vi "RT Driver VI.vi"(7 "Operation":T1, 11 "Device Reference in":T2 format="%.0x") -> (0 "Error Code":i32)   [LabVIEW 2015, in "J1939 Addon Engine.lvlib"]
uses:
  J1939 Addon Engine.lvlib
  <vilib>/NI Veristand/Custom Device API/Custom Device Item Ref.ctl
  <vilib>/NI Veristand/Custom Device API/Hardware Interface Driver VI Operation.ctl
  <vilib>/NI/NIVS Inline Async API/_VS Inline Async API/VS Inline Async API/VS Inline Async API.lvclass/VS Inline Async API.ctl
  <vilib>/NI/NIVS Inline Async API/_Data Access Engine/Data Access Engine/Data Access Engine.lvclass/Data Access Engine.ctl
  <vilib>/NI/NIVS Inline Async API/_Data Access Engine/Access Type Classes/Write/Write.lvclass/Write.ctl
  <vilib>/NI/NIVS Inline Async API/_Data Access Engine/Access Type Classes/ReadWrite/ReadWrite.lvclass/ReadWrite.ctl
  <vilib>/NI/NIVS Inline Async API/_Data Access Engine/Access Type Classes/Read/Read.lvclass/Read.ctl
  <vilib>/NI/NIVS Inline Async API/_Data Access Engine/Data Access Engine/Methods/Data.Engine.Read Data from HW.vi
  <vilib>/NI/NIVS Inline Async API/_VS Inline Async API/Error Handling Process/SubVIs/Error.GetError.vi
  <vilib>/NI Veristand/Custom Device API/NI VeriStand - Set Channel Values by Block Data Reference.vi
  <vilib>/NI Veristand/Custom Device API/NI VeriStand - Get Channel Values by Block Data Reference.vi
  <vilib>/NI/NIVS Inline Async API/_Data Access Engine/Data Access Engine/Methods/Data.Engine.Write Data to HW.vi
  <vilib>/NI/NIVS Inline Async API/_Data Access Engine/Access Type Classes/ReadWrite/ReadWrite.EngineData.vi
  <vilib>/NI/NIVS Inline Async API/_Data Access Engine/Access Type Classes/Write/Write.EngineData.vi
  <vilib>/NI/NIVS Inline Async API/_Data Access Engine/Access Type Classes/Read/Read.EngineData.vi
  <vilib>/NI Veristand/Custom Device API/NI VeriStand - Get Channel Value by Data Reference.vi
  <vilib>/NI Veristand/Custom Device API/NI VeriStand - Set Channel Value by Data Reference.vi
  SubVIs/Main.Load 986x Bitfile.vi
  SubVIs/Main.InitializeXNET.vi
  <vilib>/NI Veristand/Custom Device API/Global Data Refs.vi
  <vilib>/xnet/xnet.llb/XNET Read.vi
  <vilib>/xnet/xnet.llb/XNET Read (Signal Single-point).vi
  <vilib>/xnet/xnet.llb/XNET Read (Signal XY).vi
  <vilib>/xnet/xnet.llb/XNET Write.vi
  <vilib>/xnet/xnet.llb/XNET Write (Signal Single-point).vi
  <vilib>/xnet/xnet.llb/XNET Start.vi
  <vilib>/xnet/xnet.llb/XNET Stop.vi
  <vilib>/NI/NIVS Inline Async API/_VS Inline Async API/VS Inline Async API/VS Inline Async API.lvclass
  <vilib>/NI Veristand/Custom Device Tools/Custom Device Utility Library/Custom Device Utility Library.lvlib
  <vilib>/NI VeriStand/Custom Device API/Custom Device API.lvlib
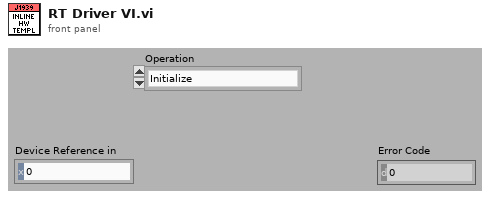
[diagram p1: front panel]
types:
  T1 = typedef "Custom Device API.lvlib/Hardware Interface Driver VI Operation.ctl" = enum16{"Initialize", "Start", "Read Data from HW", "Write Data to HW", "Close"}
  T2 = typedef "Custom Device API.lvlib/Custom Device Item Ref.ctl" = u64
  T3 = typedef "J1939 Addon Engine.lvlib/Main.State Variables.ctl" = cluster{"Main App":T4, "Protocol App":T5}
  T4 = typedef "J1939 Addon Engine.lvlib/Main.Settings.ctl" = cluster{"Device Error":errorcluster, "FPGA Session":u32, "Incoming Decimation":u32, "Outgoing Decimation":u32, "Process":refnum<class "VS Inline Async API.lvclass">}
  T5 = typedef "J1939 Addon Engine.lvlib/Protocol.App Settings.ctl" = cluster{"XNET Settings":T6, "Data":T7[], "DTCs":T13[], "Sim Addresses LUT":variant, "Data Table LUT":variant, "MonitorTool.Network":T8, "Name":string}
  T6 = typedef "J1939 Addon Shared.lvlib/XNET Settings.ctl" = cluster{"Database":refnum<k21>, "Cluster":refnum<k21>, "Port":string, "Baud rate [Bd]":u32, "Termination":u32, "Incoming Rate":u32, "Outcoming Rate":u32, "Write Decimation":u32}
  T7 = typedef "J1939 Addon Engine.lvlib/Protocol.XNET Refs.ctl" = cluster{"Network":T8, "Incoming.Use":bool, "Incoming.Session":refnum<k21>, "Incoming.Refs":T9[], "Incoming.Values":dbl[], "Outgoing.Frames":T11[], "Outgoing.Initialize":bool, "Outgoing.Refs":T9[], "Outgoing.Values":dbl[], "RequestDataTable":refnum<k33>, "Timing.Use":bool, "Timing.Index":i32[], "Timing.Refs":T9[], "Timing.Values":dbl[], "Disable.Refs":T9[], "Disable.Values":dbl[], "Trigger.Refs":T9[], "Trigger.Values":dbl[]}
  T8 = typedef "J1939 Addon Shared.lvlib/Monitor Settings.ctl" = cluster{"Address":u8, "Name":u64}
  T9 = typedef "Custom Device API.lvlib/Block Data Reference.ctl" = cluster{"Data Reference":T10, "Offset":u64, "Length":u64}
  T10 = typedef "Custom Device API.lvlib/Data Reference.ctl" = i32
  T11 = typedef "J1939 Addon Engine.lvlib/Main.Outgoing.Frame.Settings.ctl" = cluster{"Offset":u32, "Length":u32, "Cyclic?":bool, "Disable.Index":i32, "Disable?":bool, "Trigger":T12, "Trigger.Index":i32, "XNET Session":refnum<k21>}
  T12 = typedef "J1939 Addon Shared.lvlib/Outgoing Event Trigger Types.ctl" = enum16{"Channel value change", "Trigger channel (not zero)", "Channel value change or trigger channel (not zero)", "Trigger channel (any value change)", "Channel value change or trigger channel (any value change)"}
  T13 = typedef "J1939 Addon Engine.lvlib/Engine.DTC Settings.ctl" = cluster{"Data":T14, "FIFOs":T15}
  T14 = typedef "J1939 Addon Shared.lvlib/Compiled Simulated Settings.ctl" = cluster{"DM1 Ref":T9[], "DM1 Value":dbl[], "DM1 Enable Ref":T9[], "DM1 Enable Value":dbl[], "DM2 Ref":T9[], "DM2 Value":dbl[], "DM2 Enable Ref":T9[], "DM2 Enable Value":dbl[]}
  T15 = typedef "J1939 Addon Engine.lvlib/Engine.DTC FIFOs.ctl" = cluster{"DM1 Data":refnum<k33>, "DM1 Enable":refnum<k33>, "DM2 Data":refnum<k33>, "DM2 Enable":refnum<k33>, "DM1 Reset":refnum<k33>, "DM2 Reset":refnum<k33>}
  T16 = typedef "J1939 Addon Shared.lvlib/Compile Addon Settings.ctl" = cluster{"XNET":T6, "Incoming Decimation":u32, "Outgoing Decimation":u32, "Bitfile":T17, "Nodes":T18, "Name":string}
  T17 = typedef "J1939 Addon Shared.lvlib/SysDef FPGA Settings.ctl" = cluster{"RT Path":path, "RIO Device":u16, "Enable":bool}
  T18 = typedef "J1939 Addon Shared.lvlib/Compiled.Node Settings.ctl" = cluster{"Monitor":T19, "Sim":T24[]}
  T19 = typedef "J1939 Addon Shared.lvlib/Compiled Monitor Tool Settings.ctl" = cluster{"Network":T8, "Data":T20}
  T20 = typedef "J1939 Addon Shared.lvlib/Device Settings.ctl" = cluster{"Incoming":T21, "Outgoing":T23}
  T21 = typedef "J1939 Addon Shared.lvlib/Incoming Settings.ctl" = cluster{"Signals":string[], "Frames":T22[], "Data.Refs":T9[], "Data.Values":dbl[], "Timing.Use":bool, "Timing.Refs":T9[], "Timing.Values":dbl[], "Timing.Index":i32[]}
  T22 = typedef "J1939 Addon Shared.lvlib/Frame Settings.ctl" = cluster{"Signals":string[], "Channel Array Position":cluster{"Offset":u32, "Length":u32}, "PGN":u32, "Cyclic?":bool, "Disable?":bool, "Disable.Index":i32, "Trigger":T12, "Trigger.Index":i32}
  T23 = typedef "J1939 Addon Shared.lvlib/Outgoing Settings.ctl" = cluster{"Frames":T22[], "Data.Refs":T9[], "Data.Values":dbl[], "Disable.Refs":T9[], "Disable.Values":dbl[], "Trigger.Refs":T9[], "Trigger.Values":dbl[]}
  T24 = typedef "J1939 Addon Shared.lvlib/Complied Simulated Device Settings.ctl" = cluster{"Network":T8, "Data":T20, "DTCs":T14}
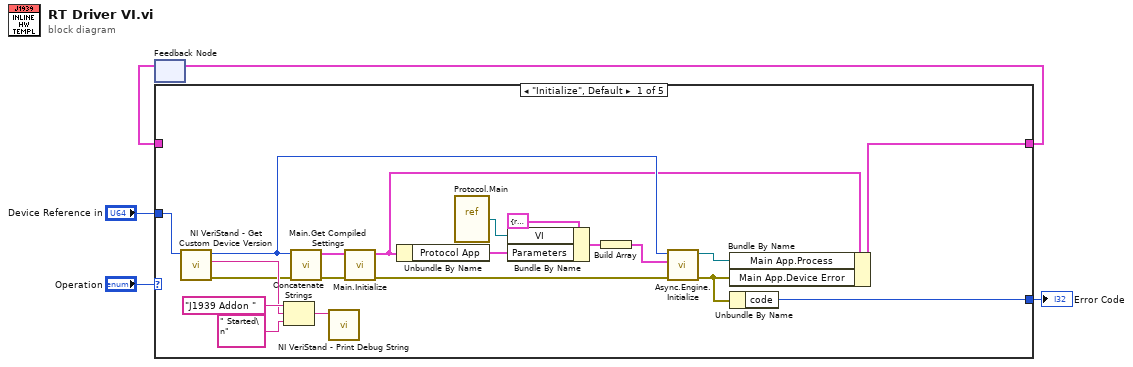
[diagram p0: block diagram]
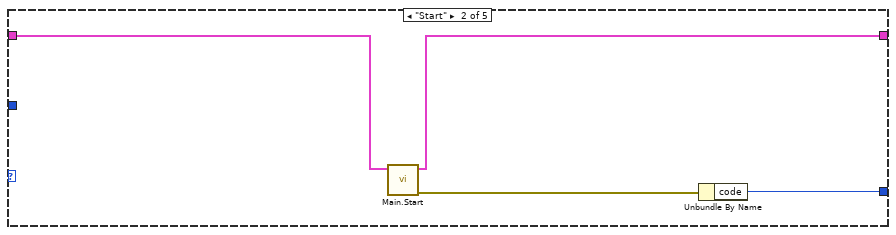
[diagram p2: hidden frame]
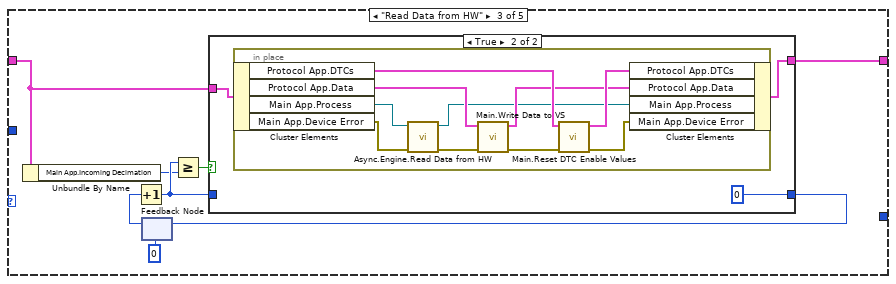
[diagram p3: hidden frame]
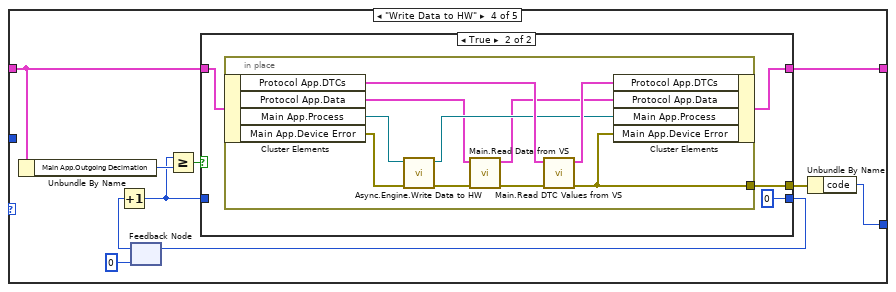
[diagram p5: hidden frame]
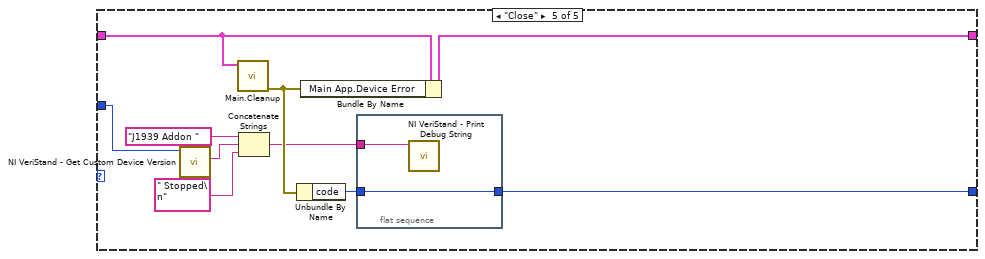
[diagram p7: hidden frame]
diagram:
  n1 = feedback #1() -> (w3:T3)  [unwired: 1 out]
  n2 = case shown="\"Initialize\", Default" "Operation" {
    tunnel: [w24 w28 w36 w62 w88] -> w4
    tunnel: w3 -> [_ w26 w37 w59 w86]
    tunnel: [w25 w29 _ w53 w79] -> w2
    tunnel: "Device Reference in" -> [w19 _ _ _ w82]
    frame "Initialize", Default {
      n3 = call <vilib>:"NI VeriStand - Get Custom Device Version.vi"("Device Ref in"=w19) -> ("error out"=w14:errorcluster, "Value"=w18:string, "Device Ref out"=w13:T2)  [unwired: 8 in]
      n4 = Concatenate Strings("J1939 Addon " ("Debug String"), w18, " Started\n" ("string")) -> (w20:string)
      n5 = call "Main.Get Compiled Settings.vi"("error in (no error)"=w14, "Item Ref in"=w13) -> ("error out"=w22:errorcluster, "Compiled"=w21:T16)  [unwired: 8 in]
      n6 = call <vilib>:"NI VeriStand - Print Debug String.vi"("Message"=w20) -> ()  [unwired: 10 in, 1 out]
      n7 = call "Main.Initialize.vi"("error in (no error)"=w22, "Compiled Settings"=w21) -> ("error out"=w16:errorcluster, "State Variables"=w7:T3)  [unwired: 8 in]
      n8 = Unbundle By Name(w7) -> ("Protocol App"=w11:T5)
      n9 = vi-ref "Protocol.Main.vi"() -> (w8:refnum<vi>)
      n10 = Bundle By Name(cluster=cluster{"VI":refnum<vi>, "Parameters":variant} {"VI"=refnum, "Parameters"=variant} ("Process"), "VI"=w8, "Parameters"=w11) -> (w9:cluster{"VI":refnum<vi>, "Parameters":variant})
      n11 = Build Array(w9) -> (w6:cluster{"VI":refnum<vi>, "Parameters":variant}[])
      n12 = call <vilib>:"Async.Engine.Initialize.vi"("error in (no error)"=w16, "Processes"=w6, "Custom Device Ref"=w13) -> ("error out"=w15:errorcluster, "Async"=w12:refnum<class "VS Inline Async API.lvclass">)  [unwired: 7 in]
      n13 = Bundle By Name(cluster=w7, "Main App.Process"=w12, "Main App.Device Error"=w15) -> (w24:T3)
      n14 = Unbundle By Name(w15) -> ("code"=w25:i32)
    }
    frame "Start" {
      n15 = call "Main.Start.vi"("State Variables in"=w26) -> ("error out"=w27:errorcluster, "State Variables out"=w28:T3)  [unwired: 9 in]
      n16 = Unbundle By Name(w27) -> ("code"=w29:i32)
    }
    frame "Read Data from HW" {
      n17 = Unbundle By Name(w37) -> ("Main App.Incoming Decimation"=w31:u32)
      n18 = feedback #2(u32 0) -> (w34:u32)
      n19 = Increment(x=w34) -> (x+1=w32:u32)
      n20 = Greater Or Equal?(x=w32, y=w31) -> (x >= y?=w33:bool)
      n21 = case shown="True" w33 {
        tunnel: w37 -> [w38 w41]
        tunnel: [w38 w40] -> w36
        tunnel: [w39 u32 0] -> w30
        tunnel: w32 -> [w39 _]
        frame False {
        }
        frame True {
          n22 = in-place {
            n23 = in-place-cluster #3(w41) -> ("Protocol App.DTCs"=w48:T13[], "Protocol App.Data"=w49:T7[], "Main App.Process"=w50:refnum<class "VS Inline Async API.lvclass">, "Main App.Device Error"=w43:errorcluster)
            n24 = call <vilib>:"Async.Engine.Read Data from HW.vi"("error in"=w43, "Async in"=w50) -> ("error out"=w52:errorcluster, "Async out"=w45:refnum<class "VS Inline Async API.lvclass">)  [unwired: 8 in]
            n25 = call "Main.Write Data to VS.vi"("error in"=w52, "Data Sessions"=w49) -> ("error out"=w51:errorcluster, "Data Sessions out"=w46:T7[])  [unwired: 8 in]
            n26 = call "Main.Reset DTC Enable Values.vi"("error in"=w51, "SimDTCs"=w48) -> ("error out"=w44:errorcluster, "SimDTCs"=w47:T13[])  [unwired: 8 in]
            n27 = in-place-cluster #3("Protocol App.DTCs"=w47, "Protocol App.Data"=w46, "Main App.Process"=w45, "Main App.Device Error"=w44) -> (w40:T3)
          }
        }
      }
      n28 = feedback-in #2(w30) -> ()
    }
    frame "Write Data to HW" {
      n29 = Unbundle By Name(w59) -> ("Main App.Outgoing Decimation"=w58:u32)
      n30 = feedback #4(u32 0) -> (w60:u32)
      n31 = Increment(x=w60) -> (x+1=w55:u32)
      n32 = Greater Or Equal?(x=w55, y=w58) -> (x >= y?=w57:bool)
      n33 = case shown="True" w57 {
        tunnel: w59 -> [w64 w67]
        tunnel: [w64 w66] -> w62
        tunnel: [w63 u32 0] -> w56
        tunnel: w55 -> [w63 _]
        tunnel: [_ w65] -> w54
        frame False {
        }
        frame True {
          n34 = in-place {
            in-place-border: [w69] -> w65
            n35 = in-place-cluster #5(w67) -> ("Protocol App.DTCs"=w78:T13[], "Protocol App.Data"=w72:T7[], "Main App.Process"=w74:refnum<class "VS Inline Async API.lvclass">, "Main App.Device Error"=w76:errorcluster)
            n36 = call <vilib>:"Async.Engine.Write Data to HW.vi"("error in (no error)"=w76, "VS Inline Async API in"=w74) -> ("error out"=w75:errorcluster, "VS Inline Async API out"=w73:refnum<class "VS Inline Async API.lvclass">)  [unwired: 8 in]
            n37 = call "Main.Read Data from VS.vi"("error in"=w75, "Data Sessions"=w72) -> ("error out"=w70:errorcluster, "Data Sessions out"=w71:T7[])  [unwired: 8 in]
            n38 = call "Main.Read DTC Values from VS.vi"("error in"=w70, "Simulated Addresses in"=w78) -> ("error out"=w69:errorcluster, "Simulated Addresses out"=w77:T13[])  [unwired: 8 in]
            n39 = in-place-cluster #5("Protocol App.DTCs"=w77, "Protocol App.Data"=w71, "Main App.Process"=w73, "Main App.Device Error"=w69) -> (w66:T3)
          }
        }
      }
      n40 = feedback-in #4(w56) -> ()
      n41 = Unbundle By Name(w54) -> ("code"=w53:i32)
    }
    frame "Close" {
      n42 = call <vilib>:"NI VeriStand - Get Custom Device Version.vi"("Device Ref in"=w82) -> ("Value"=w85:string)  [unwired: 8 in, 2 out]
      n43 = call "Main.Cleanup.vi"("State Variables"=w86) -> ("error out"=w87:errorcluster)  [unwired: 10 in]
      n44 = Concatenate Strings("J1939 Addon " ("Debug String"), w85, " Stopped\n" ("Debug String")) -> (w81:string)
      n45 = Unbundle By Name(w87) -> ("code"=w80:i32)
      n46 = Bundle By Name(cluster=w86, "Main App.Device Error"=w87) -> (w88:T3)
      n47 = flat-sequence {
        tunnel: w81 -> [w90]
        tunnel: [w89] -> w79
        tunnel: w80 -> [w89]
        frame #0 {
          n48 = call <vilib>:"NI VeriStand - Print Debug String.vi"("Message"=w90) -> ()  [unwired: 10 in, 1 out]
        }
      }
    }
  }
  "Error Code" <- w2
  n49 = feedback-in #1(w4) -> ()
